vi "main.vi"() -> ()   [LabVIEW 2013]
uses:
  <vilib>/Instr/_visa.llb/VISA Configure Serial Port (Instr).vi
panel:
  in  "baud rate":u32=115200
  in  "Com port":refnum<visa-resource-name>="COM19"
  out "XY Graph":cluster{"X":dbl, "Y":dbl}[](graph)
  in  "stop":bool
  # "Port settings"
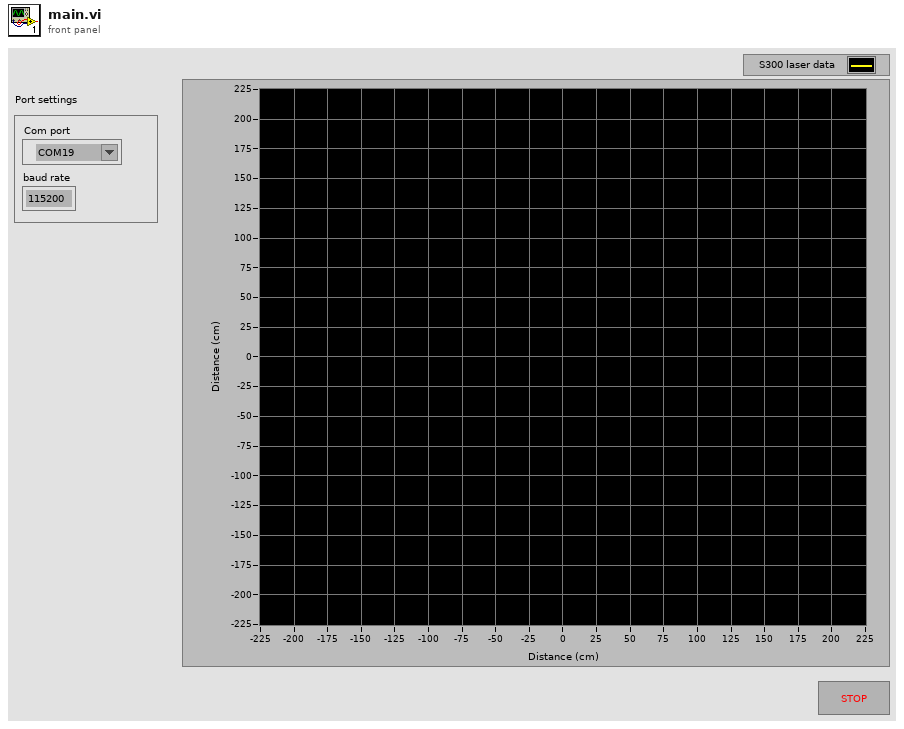
[diagram p1: front panel]
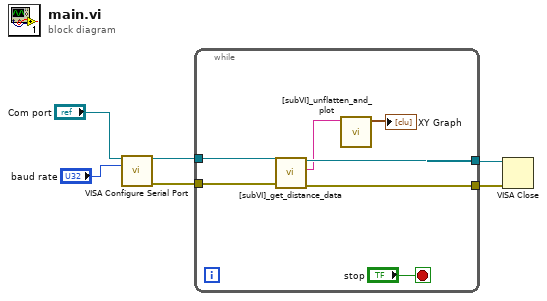
[diagram p0: block diagram]
diagram:
  n1 = call-poly "VISA Configure Serial Port"("VISA resource name"="Com port", "baud rate (9600)"="baud rate") -> ("VISA resource name out"=w4:refnum<visa-resource-name>, "error out"=w3:errorcluster)  [unwired: 12 in]
  n2 = while {
    tunnel: w4 -> [w13]
    tunnel: w3 -> [w12]
    tunnel: [w11] -> w2
    tunnel: [w10] -> w1
    stop <- "stop" stop-if-true
    n3 = call "[subVI]_get_distance_data.vi"("error in"=w12, "COM in"=w13) -> ("error out"=w10:errorcluster, "S300 data"=w8:string, "COM out"=w11:refnum<visa-resource-name>)  [unwired: 7 in]
    n4 = call "[subVI]_unflatten_and_plot.vi"("S300 data"=w8) -> ("XY Graph"=→"XY Graph":cluster{"X":dbl, "Y":dbl}[])  [unwired: 10 in]
  }
  n5 = VISA Close(VISA resource name=w2, error in (no error)=w1) -> ()  [unwired: 1 out]
